vi "get_fov_from_xml.vi"(8 "error in (no error)":errorcluster, 9 "zoom":dbl=1.0, 10 "XML string":string, 11 "TrajectoryMH100122AODRAPS in":refnum<class "TrajectoryMH100122AODRAPS.lvclass">) -> (0 "error out":errorcluster, 1 "FOVy":dbl[unit], 2 "FOVx":dbl[unit], 3 "TrajectoryMH100122AODRAPS out":refnum<class "TrajectoryMH100122AODRAPS.lvclass">)   [LabVIEW 2010, in "TrajectoryMH100122AODRAPS.lvclass"]
uses:
  TrajectoryMH100122AODRAPS.lvclass
  common/classes/XMLElement/XMLElement/XMLElement.lvclass
  TrajectoryMH100122AODRAPS.lvclass/TrajectoryMH100122AODRAPS.ctl
  common/classes/ErrorController/ErrorController/class_data.vi
  common/classes/ErrorController/ErrorController/ErrorController.lvclass
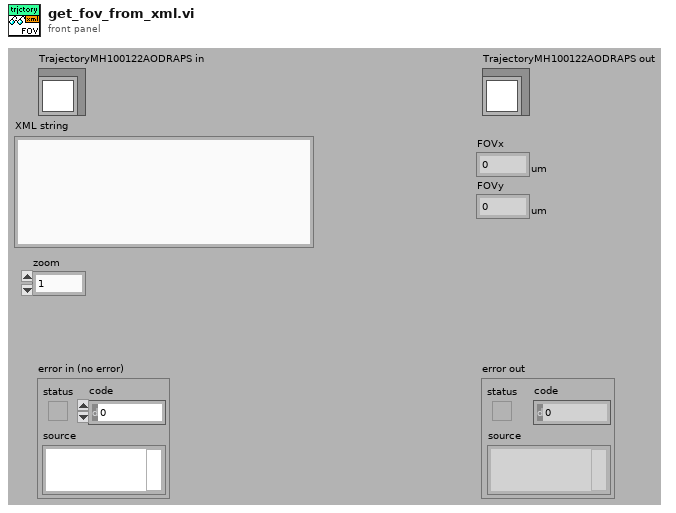
[diagram p1: front panel]
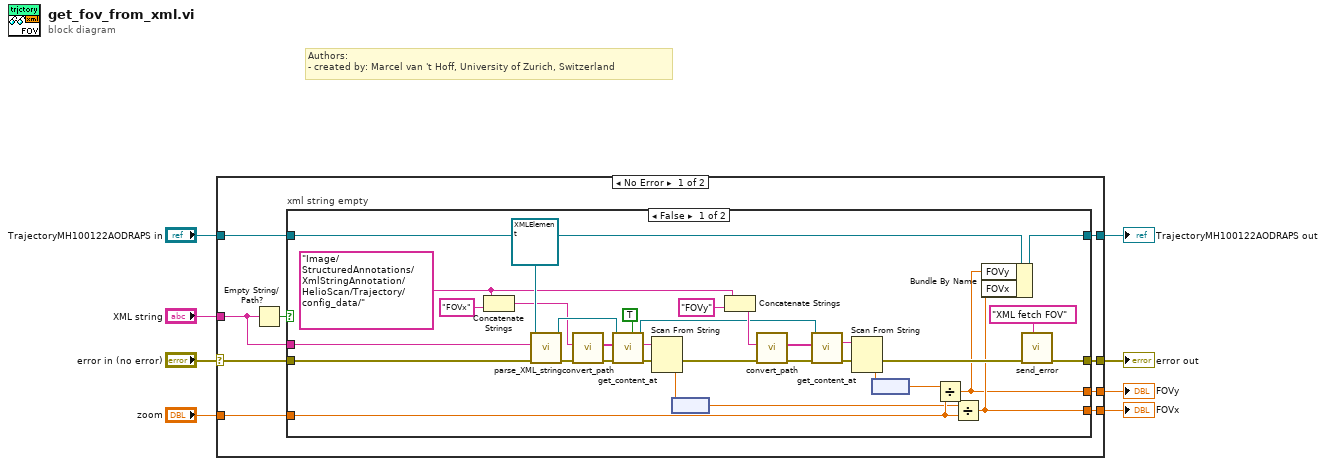
[diagram p0: block diagram]
diagram:
  # "Authors: \n- created by: Marcel van 't Hoff, University of Zurich, Switzerland"
  n1 = case shown="No Error" "error in (no error)" {
    selector: "error in (no error)" -> [w15 w54]
    tunnel: [w14 w54] -> w7
    tunnel: [w12 w53] -> w5
    tunnel: "TrajectoryMH100122AODRAPS in" -> [w13 w53]
    tunnel: "XML string" -> [w16 _]
    tunnel: [w11 _] -> w3
    tunnel: [w10 _] -> w2
    tunnel: "zoom" -> [w9 _]
    frame No Error {
      n2 = Empty String/Path?(string/path=w16) -> (empty?=w17:bool)
      n3 = case "xml string empty" shown="False" w17 {
        tunnel: w13 -> [w40 w52]
        tunnel: [w39 w52] -> w12
        tunnel: w15 -> [w38 w51]
        tunnel: [w37 w51] -> w14
        tunnel: w16 -> [w34 _]
        tunnel: [w20 _] -> w11
        tunnel: [w18 _] -> w10
        tunnel: w9 -> [w22 _]
        frame False {
          w33 = "Image/StructuredAnnotations/XmlStringAnnotation/HelioScan/Trajectory/config_data/" ("XML path zoom 2")
          n4 = Concatenate Strings(w33, "FOVx" ("string")) -> (w35:string)
          n5 = call "parse_XML_string.vi"("error in (no error)"=w38, "XML string"=w34, "Element in"=refnum<class "XMLElement.lvclass"> refnum ("XMLElement.lvclass")) -> ("error out"=w48:errorcluster, "Element out"=w47:refnum<class "XMLElement.lvclass">)  [unwired: 6 in, 1 out]
          n6 = call "convert_path.vi"("error in (no error)"=w48, "xpath in"=w35) -> ("error out"=w49:errorcluster, "key array out"=w50:string[])  [unwired: 7 in, 1 out]
          n7 = call "get_content_at.vi"("ignore IDs"=TRUE, "error in (no error)"=w49, "key chain"=w50, "Element in"=w47) -> ("error out"=w45:errorcluster, "string"=w46:string, "Element out"=w28:refnum<class "XMLElement.lvclass">)  [unwired: 4 in, 1 out]
          n8 = Scan From String(input string=w46, error in=w45) -> (error out=w26:errorcluster, output 1=w41:dbl)  [unwired: 3 in, 2 out]
          n9 = node(w41) -> (w21:dbl[unit])
          n10 = Concatenate Strings(w33, "FOVy" ("string")) -> (w31:string)
          n11 = call "convert_path.vi"("error in (no error)"=w26, "xpath in"=w31) -> ("error out"=w30:errorcluster, "key array out"=w29:string[])  [unwired: 7 in, 1 out]
          n12 = call "get_content_at.vi"("error in (no error)"=w30, "key chain"=w29, "Element in"=w28) -> ("error out"=w27:errorcluster, "string"=w23:string)  [unwired: 5 in, 2 out]
          n13 = Scan From String(input string=w23, error in=w27) -> (error out=w25:errorcluster, output 1=w24:dbl)  [unwired: 3 in, 2 out]
          n14 = node(w24) -> (w19:dbl[unit])
          n15 = Divide(x=w19, y=w22) -> (x/y=w18:dbl[unit])
          n16 = Divide(x=w21, y=w22) -> (x/y=w20:dbl[unit])
          n17 = Bundle By Name(cluster=w40, "FOVy"=w18, "FOVx"=w20) -> (w39:refnum<class "TrajectoryMH100122AODRAPS.lvclass">)
          n18 = call "send_error.vi"("additional message"="XML fetch FOV", "error in (no error)"=w25) -> ("error out"=w37:errorcluster)  [unwired: 9 in]
        }
        frame True {
        }
      }
    }
    frame Error {
    }
  }
  "error out" <- w7
  "TrajectoryMH100122AODRAPS out" <- w5
  "FOVx" <- w3
  "FOVy" <- w2
